vi "get_z_voltage.vi"(8 "error in":errorcluster, 11 "PZT in":refnum<class "PZT.lvclass">) -> (0 "error out":errorcluster, 2 "Z Voltage out":i16, 3 "PZT out":refnum<class "PZT.lvclass">)   [LabVIEW 2020, in "PZT.lvclass"]
uses:
  PZT.lvclass
  PZT.lvclass/PZT.ctl
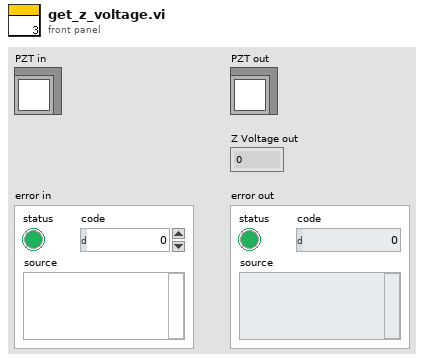
[diagram p1: front panel]
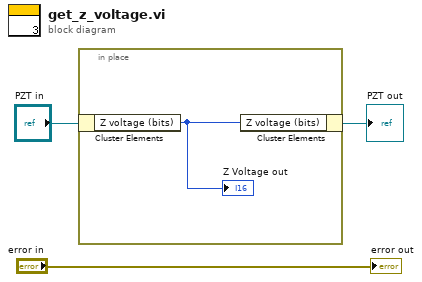
[diagram p0: block diagram]
diagram:
  n1 = in-place {
    n2 = in-place-cluster #1("PZT in") -> ("Z voltage (bits)"=w4:i16)
    "Z Voltage out" <- w4
    n3 = in-place-cluster #1("Z voltage (bits)"=w4) -> (→"PZT out":refnum<class "PZT.lvclass">)
  }
  "error out" <- "error in"
